vi "TIFF Set File Name.vi"(8 "error in (no error)":errorcluster, 10 "para1":cluster{}, 11 "para0":cluster{}) -> (0 "error out":errorcluster, 2 "function return":i8, 3 "para0 out":cluster{})   [LabVIEW 2018]
doc: "LIBTIFF_DLL_IMPEXP const char* TIFFSetFileName(TIFF*, const char *);\nextern const char* TIFFSetFileName(TIFF*, const char *);"
uses:
  libtiff3.dll
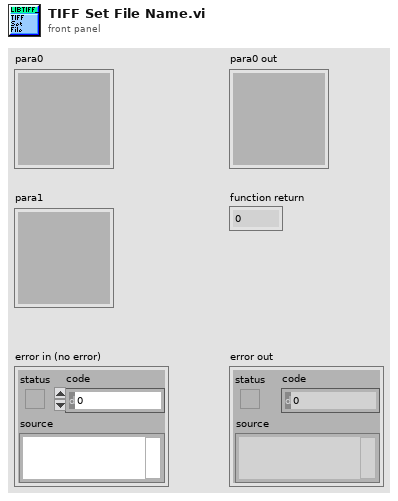
[diagram p1: front panel]
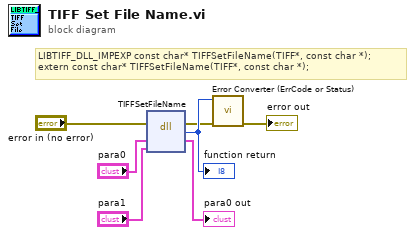
[diagram p0: block diagram]
diagram:
  # "LIBTIFF_DLL_IMPEXP\tconst char* TIFFSetFileName(TIFF*, const char *);\nextern\tconst char* TIFFSetFileName(TIFF*, const char *);"
  n1 = dll-call lib="C:/Users/johan/Downloads/LabVIEW software/LabVIEW software/IX-81 Software/lib/tiff/LibTiffLabview/libtiff3.*" fn="TIFFSetFileName"(error in="error in (no error)", "para0"="para0", "para1"="para1") -> (error out=w2:errorcluster, w7:i8, "para0"=→"para0 out":cluster{})  [unwired: 3 in, 1 out]
  "function return" <- w7
  n2 = call "Error Converter (ErrCode or Status).vi"("error in (no error)"=w2, "error code"=w7) -> ("error out"=→"error out":errorcluster)  [unwired: 9 in]
